vi "3-5 my_LED_step4.vi"() -> ()   [LabVIEW 2014]
doc: "------------------------------------\nAuther: Koji Ohashi\nCopyright (c) 2020 Japan LabVIEW Users Group, Volunteer members.\nThis VI is released under the MIT License.\nhttp://opensource.org/licenses/mit-license.php\n------------------------------------"
panel:
  out "Current (mA)":dbl
  in  "Power-supply voltage (V)":enum16{"1.8 V", "3.3 V", "5 V"}(ring)=enum."5 V"
  in  "stop":bool
  out "LED Broken":bool
  in  "Continuous Forward Current (mA)":dbl=30.0
  out "Current (A)":dbl
  in  "Current Limiting Resistor (Ω)":dbl=300.0
  in  "Forward Voltage (V)":dbl=1.2 min=0.0 step=0.1
  out "Voltage (V)":dbl
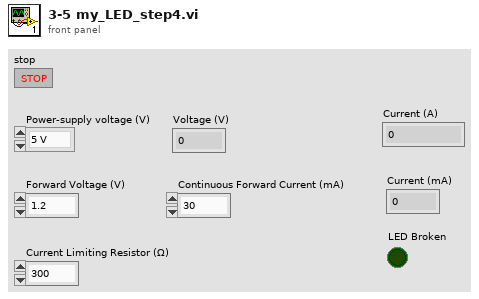
[diagram p1: front panel]
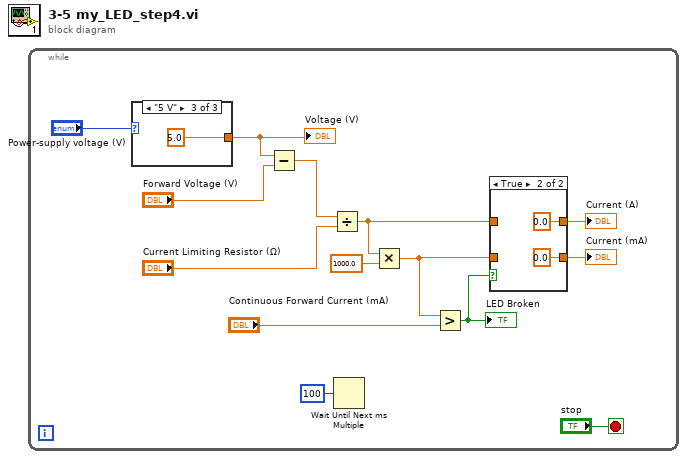
[diagram p0: block diagram]
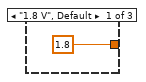
[diagram p2: hidden frame]
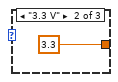
[diagram p3: hidden frame]
diagram:
  n1 = while {
    stop <- "stop" stop-if-true
    n2 = case shown="\"5 V\"" "Power-supply voltage (V)" {
      tunnel: [1.8 ("電源電圧(V)") 3.3 ("電源電圧(V)") 5.0 ("電源電圧(V)")] -> w3
      frame "1.8 V", Default {
      }
      frame "3.3 V" {
      }
      frame "5 V" {
      }
    }
    "Voltage (V)" <- w3
    n3 = Subtract(x=w3, y="Forward Voltage (V)") -> (x-y=w13:dbl)
    n4 = Divide(x=w13, y="Current Limiting Resistor (Ω)") -> (x/y=w6:dbl)
    n5 = Wait Until Next ms Multiple(millisecond multiple=u32 100) -> ()  [unwired: 1 out]
    n6 = Multiply(x=w6, y=1000.0) -> (x*y=w1:dbl)
    n7 = Greater?(x=w1, y="Continuous Forward Current (mA)") -> (0:w7:bool)
    "LED Broken" <- w7
    n8 = case shown="TRUE" w7 {
      tunnel: w6 -> [w19 _]
      tunnel: [w19 0.0] -> w5
      tunnel: [w18 0.0] -> w2
      tunnel: w1 -> [w18 _]
      frame False {
      }
      frame True {
      }
    }
    "Current (A)" <- w5
    "Current (mA)" <- w2
  }
